vi "参数设置页.vi"() -> ()   [LabVIEW 2016, in "斯坦道总氮.lvlib"]
uses:
  <vilib>/Plasmionique/MB Master/MB_Master/MB_Master.lvclass
  <vilib>/ptbypt/NI_PtbyPt.lvlib
panel:
  in  "简易流程路径":path=path "data/流程.xml"
  out "数据刷新时间":string
  in  "通讯连接":bool
  out "MB table":enum32{"Serial", "TCP"}(tab)
  in  "请选择串口:":refnum<visa-resource-name>
  in  "IP":string="127.0.0.1"
  in  "PORT":string="1001"
  in  "通信方式选择":enum16{"串口", "TCP"}(ring)
  in  "盐度自动补偿：":bool
  out "盐度补偿值":dbl caption="盐度补偿值："
  in  "刷新":bool
  in  "测量模式":T1(ring)
  in  "参数下拉列表":u16(ring) items=["总磷"=1, "总氮"=2]
  in  "量程下拉列表":enum16{"低量程", "高量程"}(ring)
  in  "测试流程路径":path=path "data/流程.xml"
  in  "标样核查量程模式":enum16{"高量程", "低量程", "自动"}(ring) caption="标样核查量程模式："
  in  "加标回收量程模式":enum16{"高量程", "低量程", "自动"}(ring) caption="加标回收量程模式："
  in  "跨度核查量程模式":enum16{"高量程", "低量程", "自动"}(ring) caption="跨度核查量程模式："
  in  "零点核查量程模式":enum16{"高量程", "低量程", "自动"}(ring) caption="零点核查量程模式："
  in  "水样测试量程模式":enum16{"高量程", "低量程", "自动"}(ring) caption="水样测试量程模式："
  out "稀释度":dbl caption="稀释度："
  out "阈值（高->低）":dbl caption="阈值（高->低）："
  out "阈值（低->高）":dbl caption="阈值（低->高）："
  out "量程下限":dbl caption="量程下限："
  out "量程上限":dbl caption="量程上限："
  out "检出限":dbl caption="检出限："
  out "曲线截距":dbl caption="曲线截距：" format="%#.6f"
  out "曲线斜率":dbl caption="曲线斜率：" format="%#.6f"
  out "二次多项式系数":dbl caption="二次多项式系数：" format="%#.6f"
  out "消解时长":dbl caption="消解时长："
  out "消解温度":dbl caption="消解温度："
  out "测量精度":u16 caption="测量精度："
  in  "标样核查标液浓度":dbl caption="标样核查标液浓度："
  in  "跨度核查标液浓度":dbl caption="跨度核查标液浓度："
  in  "零点核查标液浓度":dbl caption="零点核查标液浓度："
  in  "跨度值":dbl caption="跨度值："
  # "ppt"
  # "mg/L"
  # "mg/L"
  # "mg/L"
  # "mg/L"
  # "mg/L"
  # "min"
  # "℃"
  # "mg/L"
  # "mg/L"
  # "mg/L"
  # "mg/L"
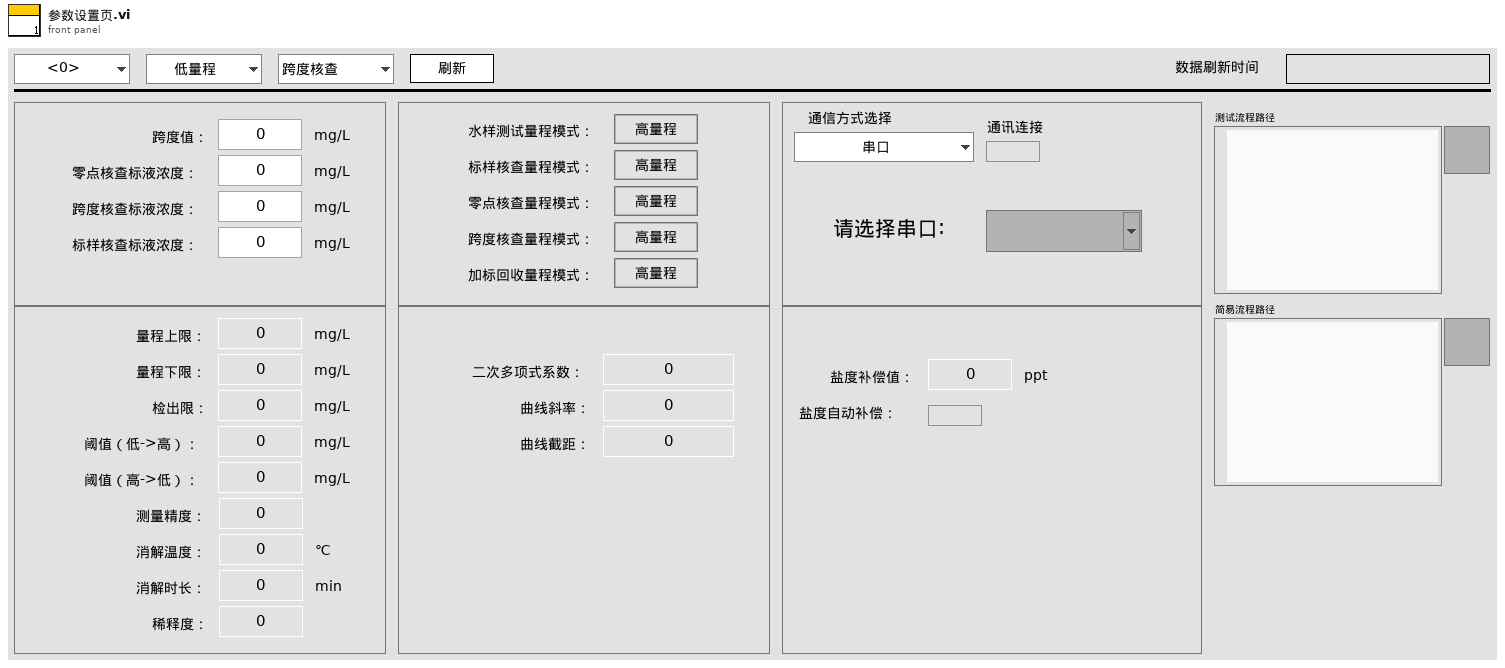
[diagram p1: front panel]
types:
  T1 = enum16{"跨度核查", "水样测量", "零点核查", "标样核查", "加标回收", "快捷测试", "空白校准", "标样校准"}
  T2 = typedef "LVStringsAndValuesArrayTypeDef_U16.ctl" = cluster{"String":string, "Value":u16}[]
  T3 = enum8{"Enabled", "Disabled", "Disabled and Grayed Out"}
  T4 = cluster{"标液浓度1":dbl, "测量吸光度1":dbl, "样品1启用":bool, "标液浓度2":dbl, "测量吸光度2":dbl, "样品2启用":bool, "标液浓度3":dbl, "测量吸光度3":dbl, "样品3启用":bool, "标液浓度4":dbl, "测量吸光度4":dbl, "样品4启用":bool, "标液浓度5":dbl, "测量吸光度5":dbl, "样品5启用":bool, "模型":enum32{"线性", "多项式"}, "精度":dbl, "XY图":cluster{"X Values":dbl[], "Y Values":dbl[]}[], "拟合公式":string, "r^2":dbl, "标样一校准时间":timestamp, "标样二校准时间":timestamp, "标样三校准时间":timestamp, "标样四校准时间":timestamp, "标样五校准时间":timestamp, "二次方程":cluster{"c":dbl, "x":dbl, "x^2":dbl}, "标定时间":timestamp}
  T5 = cluster{"系统时间":timestamp, "工作状态":u16, "测量模式":enum16{"待机", "连续模式", "周期模式", "定点模式", "受控模式", "手动模式"}, "告警代码":u16, "故障代码":u16, "日志代码":u16, "软件版本":u16, "F0":sgl, "F1":sgl, "F2":sgl, "F3":sgl, "T":sgl, "H":sgl, "id":u16, "flowid":u16, "量程":u16, "总磷控温温度1":sgl, "营养盐控温温度2":sgl, "ADC":sgl}
  T6 = cluster{"测量精度":u16, "检出限":dbl, "上限":dbl, "下限":dbl, "阈值（低->高）":dbl, "阈值（高->低）":dbl, "稀释度":dbl}
  T7 = cluster{"泵类型":u8, "进样速度":u32, "出样速度":u32, "泵阀量":u8, "光谱仪类型":u8, "光谱采样次数":u8, "氙灯次数":u8, "B":u16, "C":u16, "D":u16, "E":u16, "B_COD":u16, "C_COD":u16, "D_COD":u16, "E_COD":u16, "G":u16, "M":u16, "N":u16, "氨氮注射泵控温下限":sgl, "氨氮注射泵控温上限":sgl, "总氮注射泵控温下限":sgl, "总氮注射泵控温上限":sgl, "消解温度下限":sgl, "消解温度上限":sgl, "加热10s限值":sgl, "高温高压阀开阀温度":sgl, "总氮x公式0":u8, "总氮x公式1":sgl, "总氮x公式2":sgl, "总磷浊度稀释系数":sgl, "总磷浊度补偿权重1":sgl, "总磷浊度补偿权重2":sgl, "盐度系数":sgl, "氨氮补偿系数1":sgl, "氨氮补偿系数2":sgl}
  T8 = cluster{"标液浓度1":dbl, "测量吸光度1":dbl, "样品1启用":bool, "标液浓度2":dbl, "测量吸光度2":dbl, "样品2启用":bool, "标液浓度3":dbl, "测量吸光度3":dbl, "样品3启用":bool, "标液浓度4":dbl, "测量吸光度4":dbl, "样品4启用":bool, "标液浓度5":dbl, "测量吸光度5":dbl, "样品5启用":bool, "模型":enum32{"线性", "多项式"}, "精度":dbl, "XY图":cluster{"X Values":dbl[], "Y Values":dbl[]}[], "拟合公式":string, "r^2":dbl, "标样一校准时间":timestamp, "标样二校准时间":timestamp, "标样三校准时间":timestamp, "标样四校准时间":timestamp, "标样五校准时间":timestamp, "二次方程":cluster{"c":dbl, "x":dbl, "x^2":dbl}, "标定时间":timestamp}[][]
  T9 = typedef "斯坦道总氮.lvlib/关键参数.ctl" = cluster{"测量量程":sgl, "测量检出限":sgl, "测量精度":sgl, "测量间隔":sgl, "消解温度":sgl, "消解时长":sgl, "三项式系数":sgl, "二次多项式系数":sgl, "曲线斜率":sgl, "曲线截距":sgl, "线性相关系数":sgl, "空白校准时间":timestamp, "标样校准时间":timestamp, "测量信号值":sgl, "稀释倍数":sgl, "空白标定系数":sgl, "量程系数":sgl}
  T10 = cluster{"水样测试量程模式":enum16{"高量程", "低量程", "自动"}, "零点核查量程模式":enum16{"高量程", "低量程", "自动"}, "跨度核查量程模式":enum16{"高量程", "低量程", "自动"}, "加标回收量程模式":enum16{"高量程", "低量程", "自动"}, "标样核查量程模式":enum16{"高量程", "低量程", "自动"}}
  T11 = cluster{"总磷跨度值":dbl, "总磷零点标准液浓度":dbl, "总磷跨度标准液浓度":dbl, "总磷标准液标准浓度":dbl, "总氮跨度值":dbl, "总氮零点标准液浓度":dbl, "总氮跨度标准液浓度":dbl, "总氮标准液标准浓度":dbl, "COD跨度值":dbl, "COD零点标准液浓度":dbl, "COD跨度标准液浓度":dbl, "COD标准液标准浓度":dbl, "氨氮跨度值":dbl, "氨氮零点标准液浓度":dbl, "氨氮跨度标准液浓度":dbl, "氨氮标准液标准浓度":dbl, "磷酸盐跨度值":dbl, "磷酸盐零点标准液浓度":dbl, "磷酸盐跨度标准液浓度":dbl, "磷酸盐标准液标准浓度":dbl, "硝氮跨度值":dbl, "硝氮零点标准液浓度":dbl, "硝氮跨度标准液浓度":dbl, "硝氮标准液标准浓度":dbl, "亚硝氮跨度值":dbl, "亚硝氮零点标准液浓度":dbl, "亚硝氮跨度标准液浓度":dbl, "亚硝氮标准液标准浓度":dbl, "硫化物跨度值":dbl, "硫化物零点标准液浓度":dbl, "硫化物跨度标准液浓度":dbl, "硫化物标准液标准浓度":dbl, "硅酸盐跨度值":dbl, "硅酸盐零点标准液浓度":dbl, "硅酸盐跨度标准液浓度":dbl, "硅酸盐标准液标准浓度":dbl}
  T12 = cluster{"水样测试量程模式":u16, "零点核查量程模式":u16, "跨度核查量程模式":u16, "加标回收量程模式":u16, "标样核查量程模式":u16}
  T13 = cluster{"水样测试量程模式":enum16{"H", "L", "AUTO"}, "空白核查量程模式":enum16{"H", "L", "AUTO"}, "跨度核查量程模式":enum16{"H", "L", "AUTO"}, "加标回收量程模式":enum16{"H", "L", "AUTO"}, "标样核查量程模式":enum16{"H", "L", "AUTO"}}
  T14 = cluster{"水样测试量程模式":u16, "空白核查量程模式":u16, "跨度核查量程模式":u16, "加标回收量程模式":u16, "标样核查量程模式":u16}
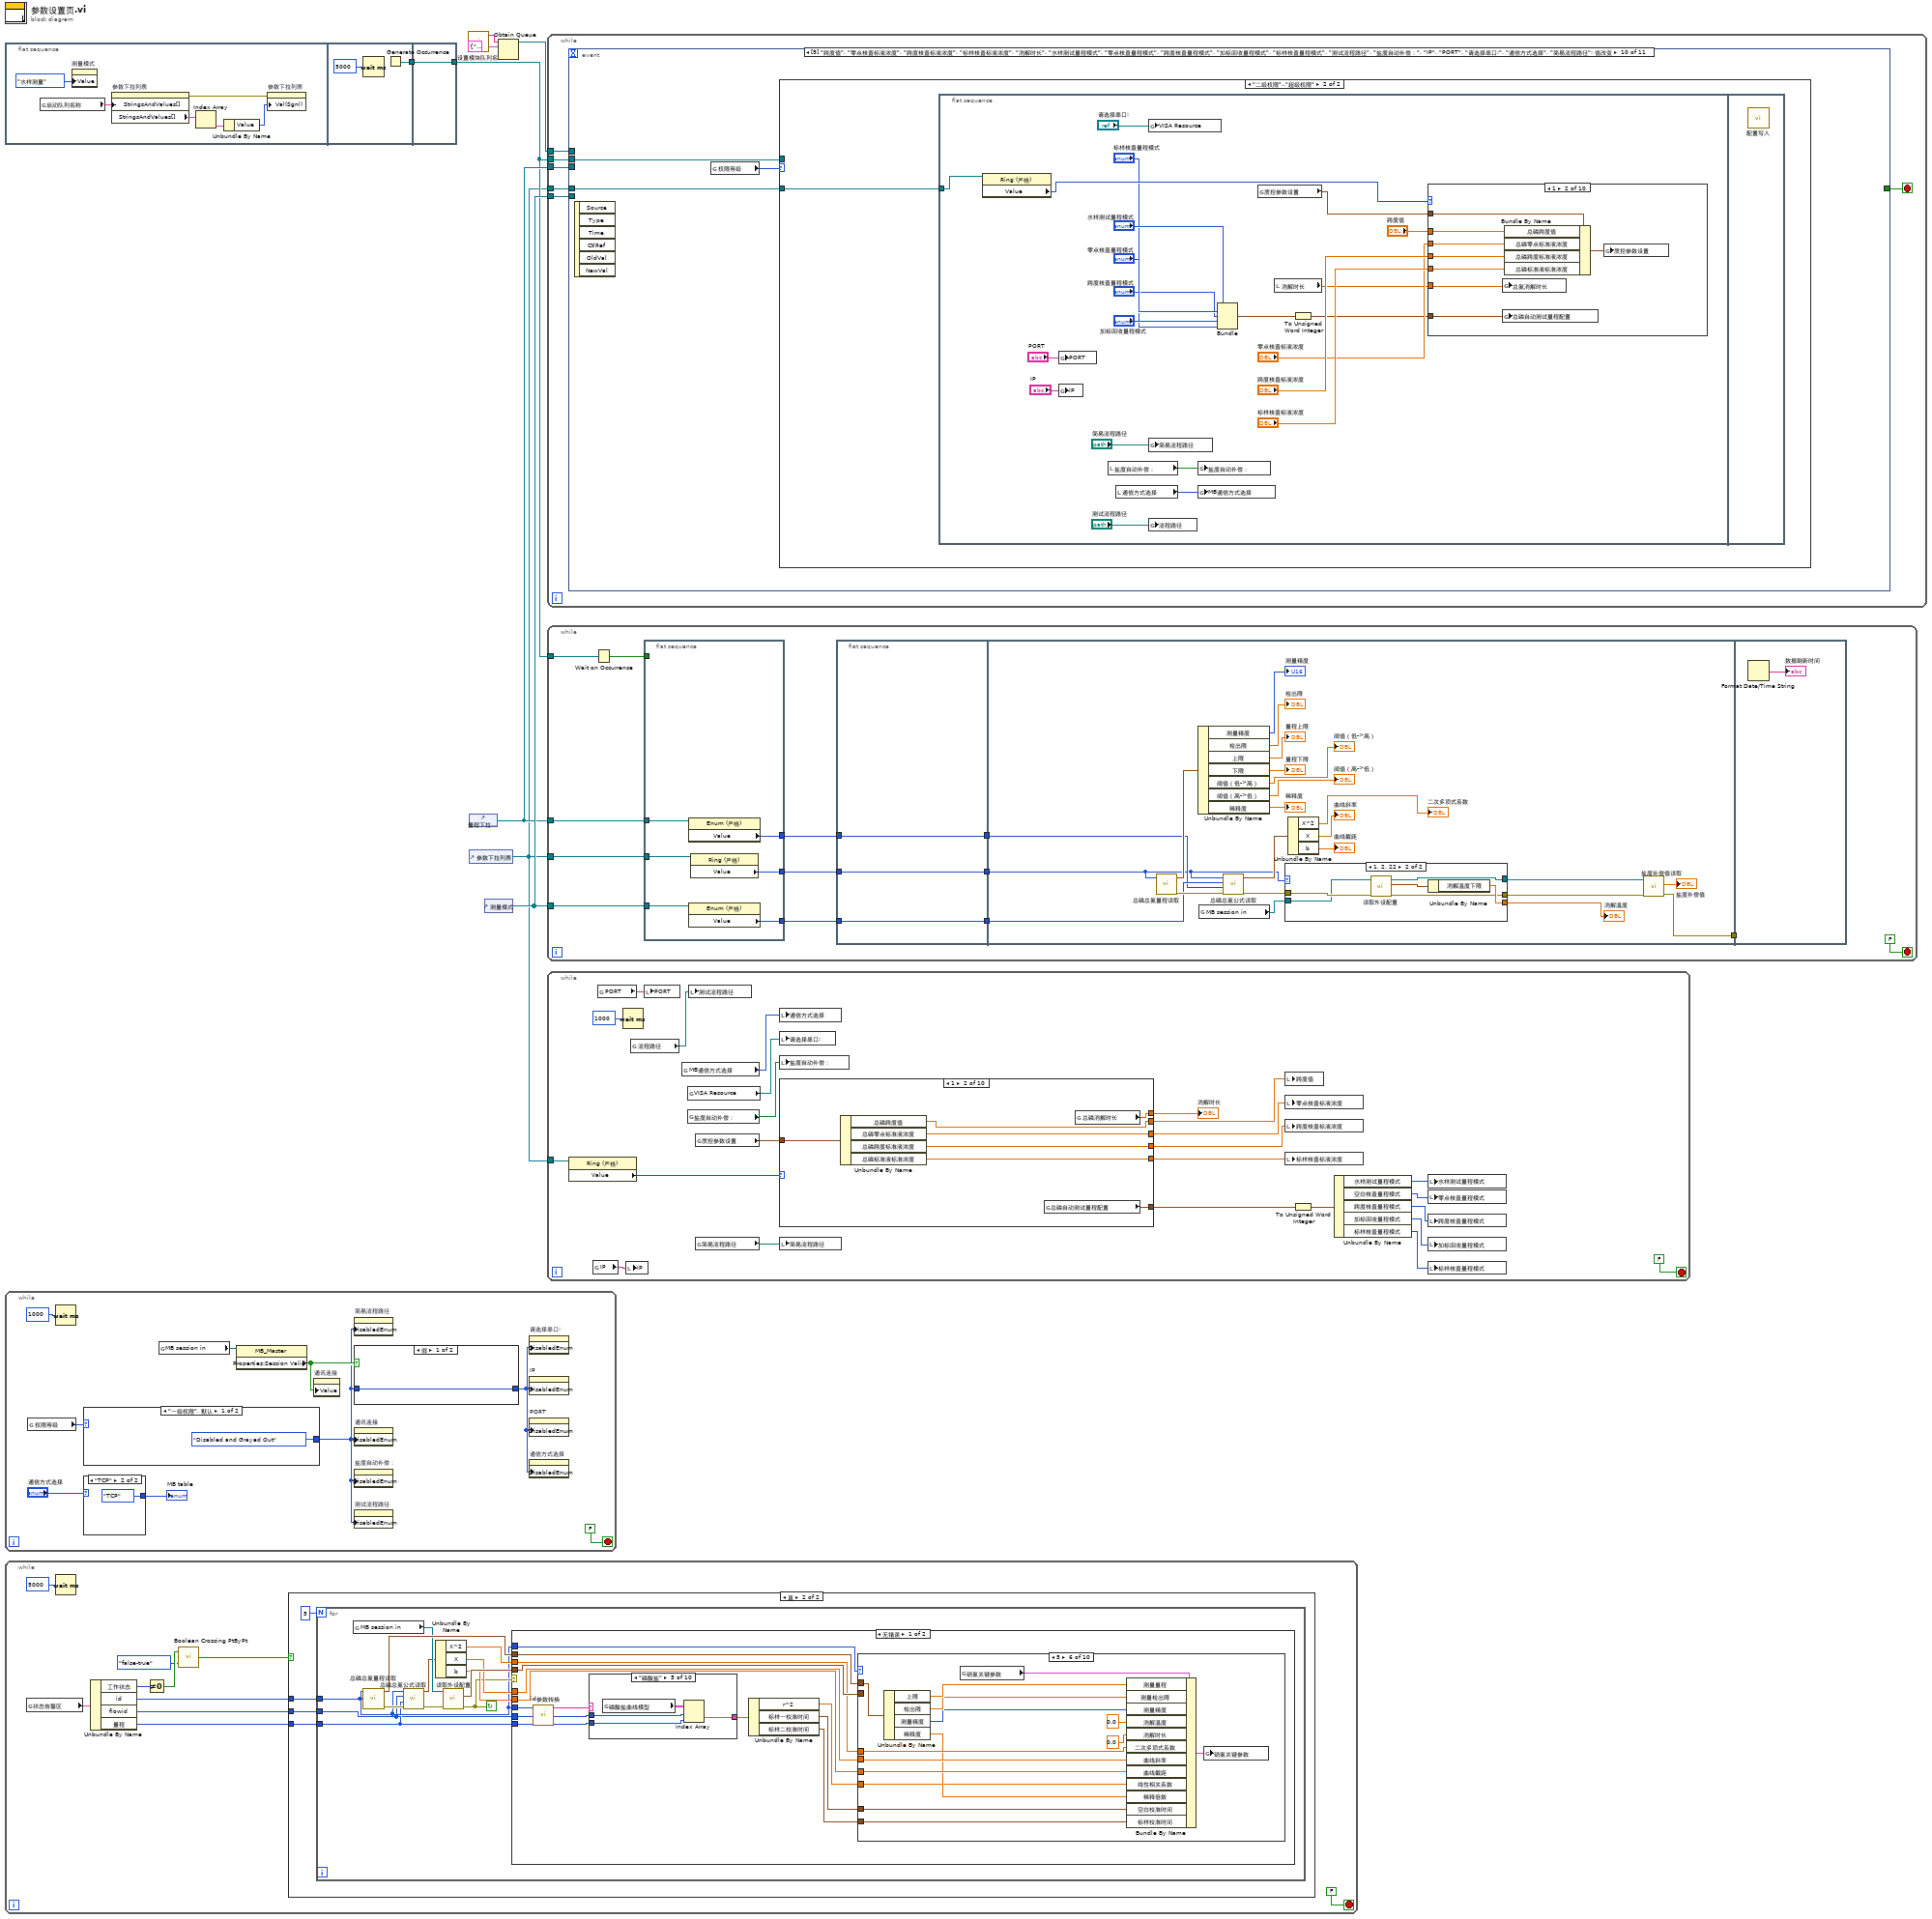
[diagram p0: block diagram]
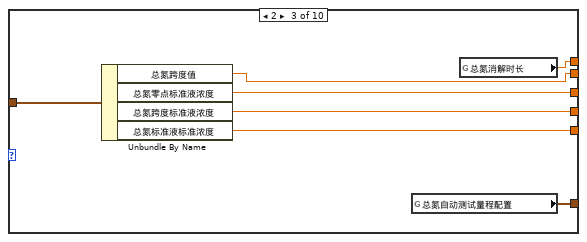
[diagram p3: hidden frame]
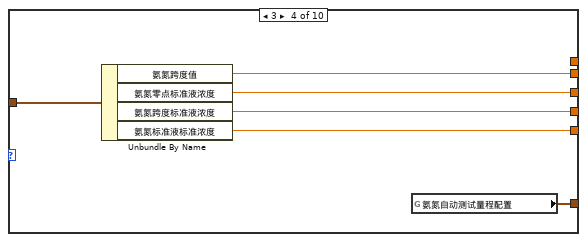
[diagram p4: hidden frame]
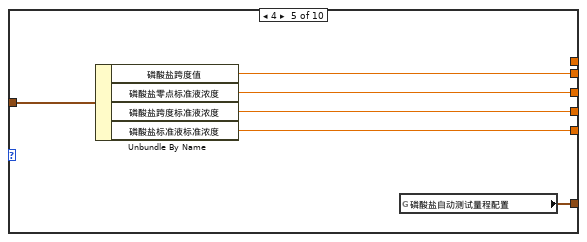
[diagram p5: hidden frame]
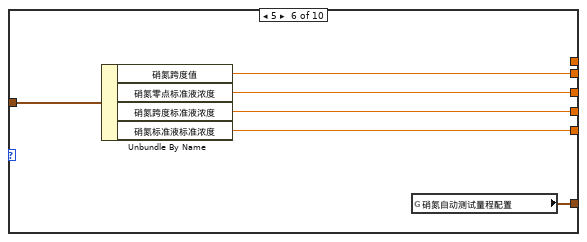
[diagram p6: hidden frame]
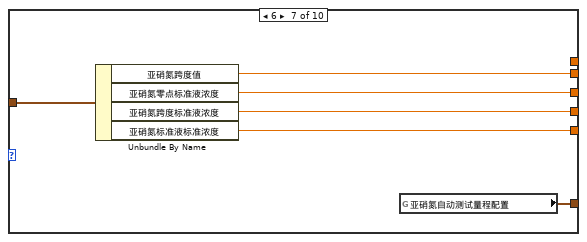
[diagram p7: hidden frame]
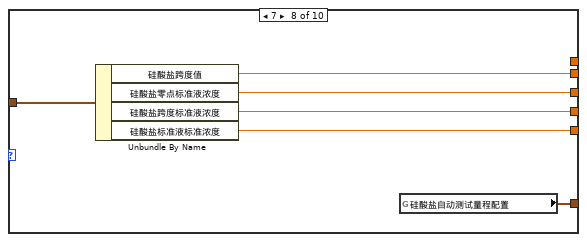
[diagram p8: hidden frame]
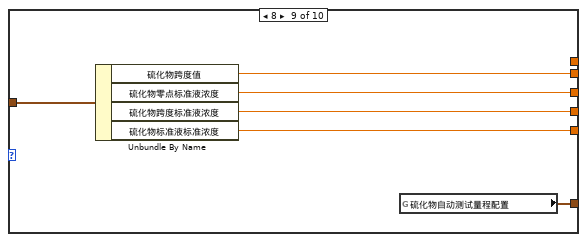
[diagram p9: hidden frame]
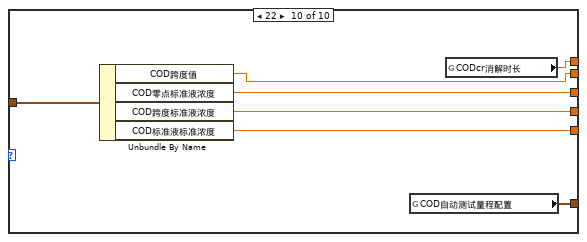
[diagram p10: hidden frame]
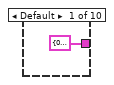
[diagram p12: hidden frame]
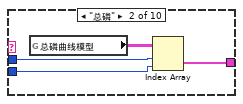
[diagram p13: hidden frame]
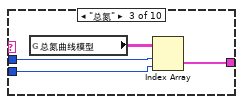
[diagram p14: hidden frame]
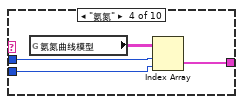
[diagram p15: hidden frame]
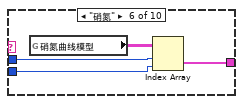
[diagram p16: hidden frame]
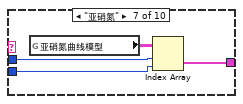
[diagram p17: hidden frame]
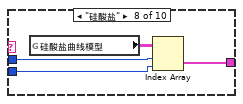
[diagram p18: hidden frame]
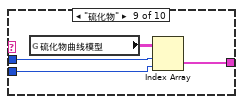
[diagram p19: hidden frame]
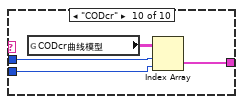
[diagram p20: hidden frame]
diagram:
  n1 = flat-sequence {
    tunnel: [w16] -> w8
    tunnel: [w17] -> w2
    tunnel: w8 -> [w17]
    frame #0 {
      n2 = global read "总磷总氮断电保存全局变量.vi" "启动队列名称"() -> (w10:cluster{"String":string, "Value":u16}[])
      n3 = property on="测量模式" class="Enum (严格)"("Value"=T1."水样测量" ("测量模式")) -> ()  [unwired: 2 in, 2 out]
      n4 = property on="参数下拉列表" class="Ring (严格)"("StringsAndValues[]"=w10) -> (error out=w13:errorcluster, "StringsAndValues[]"=w11:T2)  [unwired: 2 in, 1 out]
      n5 = Index Array(array=w11) -> (element=w12:cluster{"String":string, "Value":u16})  [unwired: 1 in]
      n6 = Unbundle By Name(w12) -> ("Value"=w14:u16)
      n7 = property on="参数下拉列表" class="Ring (严格)"(error in=w13, "Val(Sgnl)"=w14) -> ()  [unwired: 1 in, 2 out]
    }
    frame #1 {
      n8 = Wait (ms)(milliseconds to wait=u32 5000 ("等待时间（毫秒）")) -> ()  [unwired: 1 out]
      n9 = Generate Occurrence() -> (w16:refnum<k4>)
    }
    frame #2 {
    }
  }
  n10 = while {
    stop <- FALSE stop-if-true
    n11 = global read "VAR总磷总氮全局变量.vi" "权限等级"() -> (w19:enum16{"一级权限", "二级权限", "三级权限", "超级权限"})
    n12 = Wait (ms)(milliseconds to wait=u32 1000 ("等待时间（毫秒）")) -> ()  [unwired: 1 out]
    n13 = case shown="\"一级权限\", 默认" w19 {
      tunnel: [T3."Disabled and Grayed Out" ("禁用") T3."Enabled" ("禁用")] -> w18
      frame "一级权限", Default {
      }
      frame "二级权限".."超级权限" {
      }
    }
    n14 = case shown="\"TCP\"" "通信方式选择" {
      tunnel: [enum32{"Serial", "TCP"}."Serial" ("MB table") enum32{"Serial", "TCP"}."TCP" ("MB table")] -> w21
      frame "串口", Default {
      }
      frame "TCP" {
      }
    }
    "MB table" <- w21
    n15 = global read "VAR总磷总氮全局变量.vi" "MB session in"() -> (w25:refnum<class "MB_Master.lvclass">)
    n16 = property class="MB_Master"(reference=w25) -> ("Properties:Session Valid"=w23:bool)  [unwired: 1 in, 2 out]
    n17 = property on="通讯连接" class="Bool (严格)"("Value"=w23) -> ()  [unwired: 2 in, 2 out]
    n18 = property on="简易流程路径" class="Path"("DisabledEnum"=w18) -> ()  [unwired: 2 in, 2 out]
    n19 = case shown="假" w23 {
      tunnel: [w31 T3."Disabled and Grayed Out" ("禁用")] -> w22
      tunnel: w18 -> [w31 _]
      frame False {
      }
      frame True {
      }
    }
    n20 = property on="通讯连接" class="Bool (严格)"("DisabledEnum"=w18) -> ()  [unwired: 2 in, 2 out]
    n21 = property on="盐度自动补偿：" class="Bool (严格)"("DisabledEnum"=w18) -> ()  [unwired: 2 in, 2 out]
    n22 = property on="测试流程路径" class="Path"("DisabledEnum"=w18) -> ()  [unwired: 2 in, 2 out]
    n23 = property on="请选择串口:" class="VISAName"("DisabledEnum"=w22) -> ()  [unwired: 2 in, 2 out]
    n24 = property on="IP" class="Str"("DisabledEnum"=w22) -> ()  [unwired: 2 in, 2 out]
    n25 = property on="PORT" class="Str"("DisabledEnum"=w22) -> ()  [unwired: 2 in, 2 out]
    n26 = property on="通信方式选择" class="Enum (严格)"("DisabledEnum"=w22) -> ()  [unwired: 2 in, 2 out]
  }
  n27 = while {
    stop <- FALSE stop-if-true
    n28 = global read "VAR总磷总氮全局变量.vi" "状态告警区"() -> (w42:T5)
    n29 = Wait (ms)(milliseconds to wait=u32 5000 ("等待时间（毫秒）")) -> ()  [unwired: 1 out]
    n30 = Unbundle By Name(w42) -> ("工作状态"=w38:u16, "id"=w39:u16, "flowid"=w40:u16, "量程"=w41:u16)
    n31 = Not Equal To 0?(x=w38) -> (x != 0?=w37:bool)
    n32 = call <vilib>:"Boolean Crossing PtByPt.vi"("direction"=enum16{"either", "false-true", "true-false"}."false-true", "input"=w37) -> ("crossing"=w35:bool)  [unwired: 1 in]
    n33 = case shown="真" w35 {
      tunnel: w41 -> [_ w46]
      tunnel: w40 -> [_ w45]
      tunnel: w39 -> [_ w44]
      frame False {
      }
      frame True {
        n34 = for {
          N: 5 -> [_]
          tunnel: w46 -> [w48]
          tunnel: w45 -> [w47]
          tunnel: w44 -> [w49]
          stop <- w50 continue-if-true
          n35 = global read "VAR总磷总氮全局变量.vi" "MB session in"() -> (w58:refnum<class "MB_Master.lvclass">)
          n36 = call "总磷总氮量程读取.vi"("测量参数"=w49) -> ("error out"=w52:errorcluster, "量程参数读取"=w59:T6)  [unwired: 9 in]
          n37 = call "总磷总氮公式读取.vi"("error in (no error)"=w52, "量程"=w48, "测量模式"=w47, "测量参数"=w49) -> ("error out"=w51:errorcluster, "公式"=w56:cluster{"X^2":dbl, "X":dbl, "b":dbl})  [unwired: 6 in]
          n38 = Unbundle By Name(w56) -> ("X^2"=w55:dbl, "X"=w54:dbl, "b"=w53:dbl)
          n39 = call "读取外设配置.vi"("error in (no error)"=w51, "MB session in"=w58) -> ("error out"=w50:errorcluster, "外设配置"=w57:T7)  [unwired: 7 in, 1 out]
          n40 = case shown="无错误" w50 {
            tunnel: w59 -> [w73 _]
            tunnel: w57 -> [w72 _]
            tunnel: w55 -> [w71 _]
            tunnel: w54 -> [w70 _]
            tunnel: w53 -> [w69 _]
            tunnel: w49 -> [w68 _]
            tunnel: w49 -> [w65 _]
            tunnel: w48 -> [w61 _]
            tunnel: w47 -> [w60 _]
            frame No Error {
              n41 = call "id参数转换.vi"("id"=w65) -> ("table输出"=w67:string)  [unwired: 9 in, 1 out]
              n42 = case shown="\"磷酸盐\"" w67 {
                tunnel: w61 -> [_ w77 w79 w84 w88 w92 w96 w100 w104 w108]
                tunnel: w60 -> [_ w78 w80 w85 w89 w93 w97 w101 w105 w109]
                tunnel: [T4 {"标液浓度1"=0.0, "测量吸光度1"=0.0, "样品1启用"=FALSE, "标液浓度2"=0.0, "测量吸光度2"=0.0, "样品2启用"=FALSE, "标液浓度3"=0.0, "测量吸光度3"=0.0, "样品3启用"=FALSE, "标液浓度4"=0.0, "测量吸光度4"=0.0, "样品4启用"=FALSE, "标液浓度5"=0.0, "测量吸光度5"=0.0, "样品5启用"=FALSE, "模型"=enum."线性", "精度"=0.0, "XY图"=[], "拟合公式"="", "r^2"=0.0, "标样一校准时间"=timestamp(0 s since 1904-01-01), "标样二校准时间"=timestamp(0 s since 1904-01-01), "标样三校准时间"=timestamp(0 s since 1904-01-01), "标样四校准时间"=timestamp(0 s since 1904-01-01), "标样五校准时间"=timestamp(0 s since 1904-01-01), "二次方程"={"c"=0.0, "x"=0.0, "x^2"=0.0}, "标定时间"=timestamp(0 s since 1904-01-01)} ("总磷曲线模型") w75 w81 w83 w87 w91 w95 w99 w103 w107] -> w66
                frame Default {
                }
                frame "总磷" {
                  n43 = global read "校准数据全局变量.vi" "总磷曲线模型"() -> (w76:T8)
                  n44 = Index Array(array=w76, index (row)=w78, index (col)=w77) -> (element=w75:T4)
                }
                frame "总氮" {
                  n45 = global read "校准数据全局变量.vi" "总氮曲线模型"() -> (w82:T8)
                  n46 = Index Array(array=w82, index (row)=w80, index (col)=w79) -> (element=w81:T4)
                }
                frame "氨氮" {
                  n47 = global read "校准数据全局变量.vi" "氨氮曲线模型"() -> (w86:T8)
                  n48 = Index Array(array=w86, index (row)=w85, index (col)=w84) -> (element=w83:T4)
                }
                frame "磷酸盐" {
                  n49 = global read "校准数据全局变量.vi" "磷酸盐曲线模型"() -> (w90:T8)
                  n50 = Index Array(array=w90, index (row)=w89, index (col)=w88) -> (element=w87:T4)
                }
                frame "硝氮" {
                  n51 = global read "校准数据全局变量.vi" "硝氮曲线模型"() -> (w94:T8)
                  n52 = Index Array(array=w94, index (row)=w93, index (col)=w92) -> (element=w91:T4)
                }
                frame "亚硝氮" {
                  n53 = global read "校准数据全局变量.vi" "亚硝氮曲线模型"() -> (w98:T8)
                  n54 = Index Array(array=w98, index (row)=w97, index (col)=w96) -> (element=w95:T4)
                }
                frame "硅酸盐" {
                  n55 = global read "校准数据全局变量.vi" "硅酸盐曲线模型"() -> (w102:T8)
                  n56 = Index Array(array=w102, index (row)=w101, index (col)=w100) -> (element=w99:T4)
                }
                frame "硫化物" {
                  n57 = global read "校准数据全局变量.vi" "硫化物曲线模型"() -> (w106:T8)
                  n58 = Index Array(array=w106, index (row)=w105, index (col)=w104) -> (element=w103:T4)
                }
                frame "CODcr" {
                  n59 = global read "校准数据全局变量.vi" "CODcr曲线模型"() -> (w110:T8)
                  n60 = Index Array(array=w110, index (row)=w109, index (col)=w108) -> (element=w107:T4)
                }
              }
              n61 = Unbundle By Name(w66) -> ("r^2"=w64:dbl, "标样一校准时间"=w63:timestamp, "标样二校准时间"=w62:timestamp)
              n62 = case shown="5" w68 {
                tunnel: w73 -> [_ w124 w140 w155 w170 w185 w198 w213 w228 w244]
                tunnel: w72 -> [_ w120 w136 _ _ _ _ _ _ w236]
                tunnel: w71 -> [_ w117 w133 w151 w166 w181 w194 w209 w224 w240]
                tunnel: w70 -> [_ w116 w132 w150 w165 w180 w193 w208 w223 w239]
                tunnel: w69 -> [_ w115 w131 w149 w164 w179 w192 w207 w222 w238]
                tunnel: w64 -> [_ w111 w129 w145 w158 w175 _ w203 w216 w233]
                tunnel: w63 -> [_ w112 w128 w144 w160 w174 _ w202 w218 w232]
                tunnel: w62 -> [_ w113 w127 w143 w159 w173 _ w201 w217 w231]
                frame 0, Default {
                }
                frame 1 {
                  n63 = Unbundle By Name(w120) -> ("消解温度下限"=w119:sgl)
                  n64 = Unbundle By Name(w124) -> ("上限"=w123:dbl, "检出限"=w122:dbl, "测量精度"=w121:u16, "稀释度"=w114:dbl)
                  n65 = global read "VAR总磷总氮全局变量.vi" "总磷关键参数"() -> (w125:T9)
                  n66 = global read "总磷总氮断电保存全局变量.vi" "总磷消解时长"() -> (w118:dbl)
                  n67 = Bundle By Name(cluster=w125, "测量量程"=w123, "测量检出限"=w122, "测量精度"=w121, "消解温度"=w119, "消解时长"=w118, "二次多项式系数"=w117, "曲线斜率"=w116, "曲线截距"=w115, "线性相关系数"=w111, "稀释倍数"=w114, "空白校准时间"=w112, "标样校准时间"=w113) -> (w126:T9)
                  n68 = global write "VAR总磷总氮全局变量.vi" "总磷关键参数"(w126) -> ()
                }
                frame 2 {
                  n69 = Unbundle By Name(w136) -> ("消解温度下限"=w135:sgl)
                  n70 = Unbundle By Name(w140) -> ("上限"=w139:dbl, "检出限"=w138:dbl, "测量精度"=w137:u16, "稀释度"=w130:dbl)
                  n71 = global read "VAR总磷总氮全局变量.vi" "总氮关键参数"() -> (w141:T9)
                  n72 = global read "总磷总氮断电保存全局变量.vi" "总氮消解时长"() -> (w134:dbl)
                  n73 = Bundle By Name(cluster=w141, "测量量程"=w139, "测量检出限"=w138, "测量精度"=w137, "消解温度"=w135, "消解时长"=w134, "二次多项式系数"=w133, "曲线斜率"=w132, "曲线截距"=w131, "线性相关系数"=w129, "稀释倍数"=w130, "空白校准时间"=w128, "标样校准时间"=w127) -> (w142:T9)
                  n74 = global write "VAR总磷总氮全局变量.vi" "总氮关键参数"(w142) -> ()
                }
                frame 3 {
                  n75 = Unbundle By Name(w155) -> ("上限"=w154:dbl, "检出限"=w153:dbl, "测量精度"=w152:u16, "稀释度"=w148:dbl)
                  n76 = global read "VAR总磷总氮全局变量.vi" "氨氮关键参数"() -> (w156:T9)
                  n77 = Bundle By Name(cluster=w156, "测量量程"=w154, "测量检出限"=w153, "测量精度"=w152, "消解温度"=sgl 0.0, "消解时长"=sgl 0.0, "二次多项式系数"=w151, "曲线斜率"=w150, "曲线截距"=w149, "线性相关系数"=w145, "稀释倍数"=w148, "空白校准时间"=w144, "标样校准时间"=w143) -> (w157:T9)
                  n78 = global write "VAR总磷总氮全局变量.vi" "氨氮关键参数"(w157) -> ()
                }
                frame 4 {
                  n79 = Unbundle By Name(w170) -> ("上限"=w169:dbl, "检出限"=w168:dbl, "测量精度"=w167:u16, "稀释度"=w163:dbl)
                  n80 = global read "VAR总磷总氮全局变量.vi" "磷酸盐关键参数"() -> (w171:T9)
                  n81 = Bundle By Name(cluster=w171, "测量量程"=w169, "测量检出限"=w168, "测量精度"=w167, "消解温度"=sgl 0.0, "消解时长"=sgl 0.0, "二次多项式系数"=w166, "曲线斜率"=w165, "曲线截距"=w164, "线性相关系数"=w158, "稀释倍数"=w163, "空白校准时间"=w160, "标样校准时间"=w159) -> (w172:T9)
                  n82 = global write "VAR总磷总氮全局变量.vi" "磷酸盐关键参数"(w172) -> ()
                }
                frame 5 {
                  n83 = Unbundle By Name(w185) -> ("上限"=w184:dbl, "检出限"=w183:dbl, "测量精度"=w182:u16, "稀释度"=w178:dbl)
                  n84 = global read "VAR总磷总氮全局变量.vi" "硝氮关键参数"() -> (w186:T9)
                  n85 = Bundle By Name(cluster=w186, "测量量程"=w184, "测量检出限"=w183, "测量精度"=w182, "消解温度"=sgl 0.0, "消解时长"=sgl 0.0, "二次多项式系数"=w181, "曲线斜率"=w180, "曲线截距"=w179, "线性相关系数"=w175, "稀释倍数"=w178, "空白校准时间"=w174, "标样校准时间"=w173) -> (w187:T9)
                  n86 = global write "VAR总磷总氮全局变量.vi" "硝氮关键参数"(w187) -> ()
                }
                frame 6 {
                  n87 = Unbundle By Name(w198) -> ("上限"=w197:dbl, "检出限"=w196:dbl, "测量精度"=w195:u16, "稀释度"=w190:dbl)
                  n88 = global read "VAR总磷总氮全局变量.vi" "亚硝氮关键参数"() -> (w199:T9)
                  n89 = Bundle By Name(cluster=w199, "测量量程"=w197, "测量检出限"=w196, "测量精度"=w195, "消解温度"=sgl 0.0, "消解时长"=sgl 0.0, "二次多项式系数"=w194, "曲线斜率"=w193, "曲线截距"=w192, "线性相关系数"=sgl 1.0, "稀释倍数"=w190) -> (w200:T9)
                  n90 = global write "VAR总磷总氮全局变量.vi" "亚硝氮关键参数"(w200) -> ()
                }
                frame 7 {
                  n91 = Unbundle By Name(w213) -> ("上限"=w212:dbl, "检出限"=w211:dbl, "测量精度"=w210:u16, "稀释度"=w206:dbl)
                  n92 = global read "VAR总磷总氮全局变量.vi" "硅酸盐关键参数"() -> (w214:T9)
                  n93 = Bundle By Name(cluster=w214, "测量量程"=w212, "测量检出限"=w211, "测量精度"=w210, "消解温度"=sgl 0.0, "消解时长"=sgl 0.0, "二次多项式系数"=w209, "曲线斜率"=w208, "曲线截距"=w207, "线性相关系数"=w203, "稀释倍数"=w206, "空白校准时间"=w202, "标样校准时间"=w201) -> (w215:T9)
                  n94 = global write "VAR总磷总氮全局变量.vi" "硅酸盐关键参数"(w215) -> ()
                }
                frame 8 {
                  n95 = Unbundle By Name(w228) -> ("上限"=w227:dbl, "检出限"=w226:dbl, "测量精度"=w225:u16, "稀释度"=w221:dbl)
                  n96 = global read "VAR总磷总氮全局变量.vi" "硫化物关键参数"() -> (w229:T9)
                  n97 = Bundle By Name(cluster=w229, "测量量程"=w227, "测量检出限"=w226, "测量精度"=w225, "消解温度"=sgl 0.0, "消解时长"=sgl 0.0, "二次多项式系数"=w224, "曲线斜率"=w223, "曲线截距"=w222, "线性相关系数"=w216, "稀释倍数"=w221, "空白校准时间"=w218, "标样校准时间"=w217) -> (w230:T9)
                  n98 = global write "VAR总磷总氮全局变量.vi" "硫化物关键参数"(w230) -> ()
                }
                frame 22 {
                  n99 = Unbundle By Name(w236) -> ("消解温度下限"=w235:sgl)
                  n100 = Unbundle By Name(w244) -> ("上限"=w243:dbl, "检出限"=w242:dbl, "测量精度"=w241:u16, "稀释度"=w237:dbl)
                  n101 = global read "VAR总磷总氮全局变量.vi" "CODcr关键参数"() -> (w245:T9)
                  n102 = global read "总磷总氮断电保存全局变量.vi" "CODcr消解时长"() -> (w234:dbl)
                  n103 = Bundle By Name(cluster=w245, "测量量程"=w243, "测量检出限"=w242, "测量精度"=w241, "消解温度"=w235, "消解时长"=w234, "二次多项式系数"=w240, "曲线斜率"=w239, "曲线截距"=w238, "线性相关系数"=w233, "稀释倍数"=w237, "空白校准时间"=w232, "标样校准时间"=w231) -> (w246:T9)
                  n104 = global write "VAR总磷总氮全局变量.vi" "CODcr关键参数"(w246) -> ()
                }
              }
            }
            frame Error {
            }
          }
        }
      }
    }
  }
  n105 = call "设置模块队列名.vi"() -> ("Msg"=w6:string)  [unwired: 5 in]
  n106 = control-ref of="量程下拉列表"() -> (w3:refnum<vi>)
  n107 = control-ref of="参数下拉列表"() -> (w1:refnum<vi>)
  n108 = control-ref of="测量模式"() -> (w4:refnum<vi>)
  n109 = Obtain Queue(name (unnamed)=w6, element data type=cluster{"命令":string, "data":variant} {"命令"="", "data"=variant}) -> (queue out=w5:refnum<queue>)  [unwired: 3 in, 2 out]
  n110 = while {
    tunnel: w2 -> [w251]
    tunnel: w1 -> [w250]
    tunnel: w5 -> [w249]
    tunnel: w4 -> [w248]
    tunnel: w3 -> [w247]
    stop <- w252 stop-if-true
    n111 = event shown="[9] \"跨度值\", \"零点核查标液浓度\", \"跨度核查标液浓度\", \"标样核查标液浓度\", \"消解时长\", \"水样测试量程模式\", \"零点核查量程模式\", \"跨度核查量程模式\", \"加标回收量程模式\", \"标样核查量程模式\", \"测试流程路径\", \"盐度自动补偿：\", \"IP\", \"PORT\", \"请选择串口:\", \"通信方式选择\", \"简易流程路径\": 值改变" {
      selector: _ -> [_ _ _ _ _ _ _ _ _ _ _]
      dyn-events: _ -> [_ _ _ _ _ _ _ _ _ _ _]
      timeout: _ -> [_ _ _ _ _ _ _ _ _ _ _]
      tunnel: [_ TRUE _ _ _ _ _ _ _ _ _] -> w252
      tunnel: w251 -> [_ _ w254 _ _ _ _ _ _ w301 _]
      tunnel: w250 -> [_ _ _ _ w273 _ _ _ _ w303 _]
      tunnel: w249 -> [_ _ _ _ _ _ _ _ _ _ w394]
      tunnel: w248 -> [_ _ _ _ _ _ _ _ _ _ _]
      tunnel: w247 -> [_ _ _ _ _ _ _ _ _ _ _]
      event Timeout {
        n112 = event-data() -> ()  [unwired: 1 in, 3 out]
      }
      event Panel Close {
        n113 = event-data() -> ()  [unwired: 1 in, 4 out]
      }
      event "参数下拉列表", "量程下拉列表", "测量模式", "刷新": Value Change {
        n114 = event-data() -> ()  [unwired: 1 in, 6 out]
        n115 = Set Occurrence(w254) -> ()
      }
      event "跨度值", "零点核查标液浓度", "跨度核查标液浓度", "标样核查标液浓度", "消解温度", "消解时长", "检出限", "量程上限", "量程下限", "阈值（低->高）", "阈值（高->低）", "稀释度": Mouse Down {
        n116 = event-data() -> ("CtlRef"=w256:refnum<vi>)  [unwired: 1 in, 5 out]
        n117 = global read "VAR总磷总氮全局变量.vi" "权限等级"() -> (w255:enum16{"一级权限", "二级权限", "三级权限", "超级权限"})
        n118 = case shown="\"二级权限\"..\"超级权限\"" w255 {
          tunnel: w256 -> [_ w260]
          frame "一级权限", Default {
          }
          frame "二级权限".."超级权限" {
            n119 = property class="DigNum (严格)"(reference=w260) -> (reference out=w258:refnum<vi>, "Value"=w259:dbl)  [unwired: 1 in, 1 out]
            n120 = call "数字键盘.vi"("OldNumber"=w259) -> ("NewNumber"=w257:dbl)
            n121 = property class="DigNum (严格)"(reference=w258, "Val(Sgnl)"=w257) -> ()  [unwired: 1 in, 2 out]
          }
        }
      }
      event "测量精度", "检出限", "量程上限", "量程下限", "阈值（低->高）", "阈值（高->低）", "稀释度": Value Change {
        n122 = event-data() -> ()  [unwired: 1 in, 6 out]
        n123 = property class="Ring (严格)"(reference=w273) -> ("Value"=w272:u16)  [unwired: 1 in, 2 out]
        n124 = local read "阈值（低->高）"() -> (w266:dbl)
        n125 = local read "阈值（高->低）"() -> (w265:dbl)
        n126 = local read "测量精度"() -> (w263:u16)
        n127 = local read "量程下限"() -> (w268:dbl)
        n128 = local read "量程上限"() -> (w269:dbl)
        n129 = local read "稀释度"() -> (w264:dbl)
        n130 = local read "检出限"() -> (w267:dbl)
        n131 = Bundle By Name(cluster=T6 {"测量精度"=0, "检出限"=0.0, "上限"=0.0, "下限"=0.0, "阈值（低->高）"=0.0, "阈值（高->低）"=0.0, "稀释度"=0.0} ("量程参数写入"), "测量精度"=w263, "检出限"=w267, "上限"=w269, "下限"=w268, "阈值（低->高）"=w266, "阈值（高->低）"=w265, "稀释度"=w264) -> (w270:T6)
        n132 = call "总磷总氮量程写入.vi"("量程参数写入"=w270, "测量参数"=w272) -> ("error out"=w261:errorcluster)  [unwired: 8 in]
        n133 = case shown="错误" w261 {
          tunnel: ["写入成功" "写入失败"] -> w262
          frame No Error {
          }
          frame Error {
          }
        }
        n134 = One Button Dialog(message=w262) -> ()  [unwired: 1 in, 1 out]
      }
      event "消解温度": Value Change {
        n135 = event-data() -> ("NewVal"=w278:dbl)  [unwired: 1 in, 5 out]
        n136 = global read "VAR总磷总氮全局变量.vi" "MB session in"() -> (w279:refnum<class "MB_Master.lvclass">)
        n137 = call "读取外设配置.vi"("MB session in"=w279) -> ("error out"=w282:errorcluster, "外设配置"=w281:T7)  [unwired: 8 in, 1 out]
        n138 = Bundle By Name(cluster=w281, "消解温度下限"=w278) -> (w280:T7)
        n139 = call "写入外设配置.vi"("error in (no error)"=w282, "外设配置"=w280, "MB session in"=w279) -> ("error out"=w277:errorcluster)  [unwired: 7 in, 1 out]
        n140 = case shown="错误" w277 {
          tunnel: ["写入成功" "写入失败"] -> w276
          frame No Error {
          }
          frame Error {
          }
        }
        n141 = One Button Dialog(message=w276) -> ()  [unwired: 1 in, 1 out]
      }
      event "测量精度": Mouse Down {
        n142 = event-data() -> ("CtlRef"=w286:refnum<vi>)  [unwired: 1 in, 7 out]
        n143 = global read "VAR总磷总氮全局变量.vi" "权限等级"() -> (w285:enum16{"一级权限", "二级权限", "三级权限", "超级权限"})
        n144 = case shown="\"二级权限\"..\"超级权限\"" w285 {
          tunnel: w286 -> [_ w290]
          frame "一级权限", Default {
          }
          frame "二级权限".."超级权限" {
            n145 = property class="DigNum (严格)"(reference=w290) -> (reference out=w288:refnum<vi>, "Value"=w289:u16)  [unwired: 1 in, 1 out]
            n146 = call "数字键盘.vi"("OldNumber"=w289) -> ("NewNumber"=w287:dbl)
            n147 = property class="DigNum (严格)"(reference=w288, "Val(Sgnl)"=w287) -> ()  [unwired: 1 in, 2 out]
          }
        }
      }
      event "盐度补偿值": Mouse Down {
        n148 = event-data() -> ("CtlRef"=w292:refnum<vi>)  [unwired: 1 in, 3 out]
        n149 = global read "VAR总磷总氮全局变量.vi" "权限等级"() -> (w291:enum16{"一级权限", "二级权限", "三级权限", "超级权限"})
        n150 = case shown="\"二级权限\"..\"超级权限\"" w291 {
          tunnel: w292 -> [_ w294]
          frame "一级权限", Default {
          }
          frame "二级权限".."超级权限" {
            n151 = case shown="假" "盐度自动补偿：" {
              tunnel: w294 -> [w298 _]
              frame False {
                n152 = property class="DigNum (严格)"(reference=w298) -> (reference out=w296:refnum<vi>, "Value"=w297:dbl)  [unwired: 1 in, 1 out]
                n153 = call "数字键盘.vi"("OldNumber"=w297) -> ("NewNumber"=w295:dbl)
                n154 = property class="DigNum (严格)"(reference=w296, "Val(Sgnl)"=w295) -> ()  [unwired: 1 in, 2 out]
              }
              frame True {
              }
            }
          }
        }
      }
      event "盐度补偿值": Value Change {
        n155 = event-data() -> ("NewVal"=w299:dbl)  [unwired: 1 in, 5 out]
        n156 = global read "VAR总磷总氮全局变量.vi" "MB session in"() -> (w300:refnum<class "MB_Master.lvclass">)
        n157 = call "盐度补偿值写入.vi"("盐度补偿值"=w299, "MB session in"=w300) -> ()  [unwired: 8 in, 2 out]
      }
      event "跨度值", "零点核查标液浓度", "跨度核查标液浓度", "标样核查标液浓度", "消解时长", "水样测试量程模式", "零点核查量程模式", "跨度核查量程模式", "加标回收量程模式", "标样核查量程模式", "测试流程路径", "盐度自动补偿：", "IP", "PORT", "请选择串口:", "通信方式选择", "简易流程路径": Value Change {
        n158 = event-data() -> ()  [unwired: 1 in, 6 out]
        n159 = global read "VAR总磷总氮全局变量.vi" "权限等级"() -> (w302:enum16{"一级权限", "二级权限", "三级权限", "超级权限"})
        n160 = case shown="\"二级权限\"..\"超级权限\"" w302 {
          tunnel: w303 -> [_ w305]
          tunnel: w301 -> [w304 _]
          frame "一级权限", Default {
            n161 = Set Occurrence(w304) -> ()
          }
          frame "二级权限".."超级权限" {
            n162 = flat-sequence {
              tunnel: w305 -> [w326]
              frame #0 {
                n163 = property class="Ring (严格)"(reference=w326) -> ("Value"=w325:u16)  [unwired: 1 in, 2 out]
                n164 = global write "总磷总氮断电保存全局变量.vi" "PORT"("PORT") -> ()
                n165 = global write "总磷总氮断电保存全局变量.vi" "IP"("IP") -> ()
                n166 = local read "盐度自动补偿："() -> (w312:bool)
                n167 = local read "通信方式选择"() -> (w308:enum16{"串口", "TCP"})
                n168 = global write "总磷总氮断电保存全局变量.vi" "VISA Resource"("请选择串口:") -> ()
                n169 = global write "总磷总氮断电保存全局变量.vi" "简易流程路径"("简易流程路径") -> ()
                n170 = global write "总磷总氮断电保存全局变量.vi" "流程路径"("测试流程路径") -> ()
                n171 = global write "总磷总氮断电保存全局变量.vi" "盐度自动补偿："(w312) -> ()
                n172 = global write "总磷总氮断电保存全局变量.vi" "MB通信方式选择"(w308) -> ()
                n173 = Bundle("水样测试量程模式"="水样测试量程模式", "零点核查量程模式"="零点核查量程模式", "跨度核查量程模式"="跨度核查量程模式", "加标回收量程模式"="加标回收量程模式", "标样核查量程模式"="标样核查量程模式") -> (w314:T10)  [unwired: 1 in]
                n174 = global read "总磷总氮断电保存全局变量.vi" "质控参数设置"() -> (w320:T11)
                n175 = local read "消解时长"() -> (w307:dbl)
                n176 = To Unsigned Word Integer(number=w314) -> (unsigned 16bit integer=w313:T12)
                n177 = case shown="1" w325 {
                  tunnel: "跨度值" -> [_ w333 w341 w348 w355 w362 w369 w376 w383 w390]
                  tunnel: "标样核查标液浓度" -> [_ w330 w338 w345 w352 w359 w366 w373 w380 w387]
                  tunnel: "跨度核查标液浓度" -> [_ w331 w339 w346 w353 w360 w367 w374 w381 w388]
                  tunnel: "零点核查标液浓度" -> [_ w332 w340 w347 w354 w361 w368 w375 w382 w389]
                  tunnel: w320 -> [_ w335 w343 w350 w357 w364 w371 w378 w385 w392]
                  tunnel: w313 -> [_ w329 w337 w344 w351 w358 w365 w372 w379 _]
                  tunnel: w307 -> [_ w328 w336 _ _ _ _ _ _ w386]
                  frame 0, Default {
                  }
                  frame 1 {
                    n178 = global write "总磷总氮断电保存全局变量.vi" "总氮消解时长"(w328) -> ()
                    n179 = global write "总磷总氮断电保存全局变量.vi" "总磷自动测试量程配置"(w329) -> ()
                    n180 = Bundle By Name(cluster=w335, "总磷跨度值"=w333, "总磷零点标准液浓度"=w332, "总磷跨度标准液浓度"=w331, "总磷标准液标准浓度"=w330) -> (w334:T11)
                    n181 = global write "总磷总氮断电保存全局变量.vi" "质控参数设置"(w334) -> ()
                  }
                  frame 2 {
                    n182 = global write "总磷总氮断电保存全局变量.vi" "总氮消解时长"(w336) -> ()
                    n183 = global write "总磷总氮断电保存全局变量.vi" "总氮自动测试量程配置"(w337) -> ()
                    n184 = Bundle By Name(cluster=w343, "总氮跨度值"=w341, "总氮零点标准液浓度"=w340, "总氮跨度标准液浓度"=w339, "总氮标准液标准浓度"=w338) -> (w342:T11)
                    n185 = global write "总磷总氮断电保存全局变量.vi" "质控参数设置"(w342) -> ()
                  }
                  frame 3 {
                    n186 = global write "总磷总氮断电保存全局变量.vi" "氨氮自动测试量程配置"(w344) -> ()
                    n187 = Bundle By Name(cluster=w350, "氨氮跨度值"=w348, "氨氮零点标准液浓度"=w347, "氨氮跨度标准液浓度"=w346, "氨氮标准液标准浓度"=w345) -> (w349:T11)
                    n188 = global write "总磷总氮断电保存全局变量.vi" "质控参数设置"(w349) -> ()
                  }
                  frame 4 {
                    n189 = Bundle By Name(cluster=w357, "磷酸盐跨度值"=w355, "磷酸盐零点标准液浓度"=w354, "磷酸盐跨度标准液浓度"=w353, "磷酸盐标准液标准浓度"=w352) -> (w356:T11)
                    n190 = global write "总磷总氮断电保存全局变量.vi" "磷酸盐自动测试量程配置"(w351) -> ()
                    n191 = global write "总磷总氮断电保存全局变量.vi" "质控参数设置"(w356) -> ()
                  }
                  frame 5 {
                    n192 = global write "总磷总氮断电保存全局变量.vi" "硝氮自动测试量程配置"(w358) -> ()
                    n193 = Bundle By Name(cluster=w364, "硝氮跨度值"=w362, "硝氮零点标准液浓度"=w361, "硝氮跨度标准液浓度"=w360, "硝氮标准液标准浓度"=w359) -> (w363:T11)
                    n194 = global write "总磷总氮断电保存全局变量.vi" "质控参数设置"(w363) -> ()
                  }
                  frame 6 {
                    n195 = Bundle By Name(cluster=w371, "亚硝氮跨度值"=w369, "亚硝氮零点标准液浓度"=w368, "亚硝氮跨度标准液浓度"=w367, "亚硝氮标准液标准浓度"=w366) -> (w370:T11)
                    n196 = global write "总磷总氮断电保存全局变量.vi" "亚硝氮自动测试量程配置"(w365) -> ()
                    n197 = global write "总磷总氮断电保存全局变量.vi" "质控参数设置"(w370) -> ()
                  }
                  frame 7 {
                    n198 = Bundle By Name(cluster=w378, "硅酸盐跨度值"=w376, "硅酸盐零点标准液浓度"=w375, "硅酸盐跨度标准液浓度"=w374, "硅酸盐标准液标准浓度"=w373) -> (w377:T11)
                    n199 = global write "总磷总氮断电保存全局变量.vi" "硅酸盐自动测试量程配置"(w372) -> ()
                    n200 = global write "总磷总氮断电保存全局变量.vi" "质控参数设置"(w377) -> ()
                  }
                  frame 8 {
                    n201 = Bundle By Name(cluster=w385, "硫化物跨度值"=w383, "硫化物零点标准液浓度"=w382, "硫化物跨度标准液浓度"=w381, "硫化物标准液标准浓度"=w380) -> (w384:T11)
                    n202 = global write "总磷总氮断电保存全局变量.vi" "硫化物自动测试量程配置"(w379) -> ()
                    n203 = global write "总磷总氮断电保存全局变量.vi" "质控参数设置"(w384) -> ()
                  }
                  frame 22 {
                    n204 = global write "总磷总氮断电保存全局变量.vi" "CODcr消解时长"(w386) -> ()
                    n205 = Bundle By Name(cluster=w392, "COD跨度值"=w390, "COD零点标准液浓度"=w389, "COD跨度标准液浓度"=w388, "COD标准液标准浓度"=w387) -> (w391:T11)
                    n206 = global write "总磷总氮断电保存全局变量.vi" "质控参数设置"(w391) -> ()
                  }
                }
              }
              frame #1 {
                n207 = call "配置写入.vi"() -> ()  [unwired: 11 in, 1 out]
              }
            }
          }
        }
      }
      event "通讯连接": Value Change {
        n208 = event-data() -> ("NewVal"=w393:bool)  [unwired: 1 in, 5 out]
        n209 = Flush Queue(queue=w394) -> (queue out=w395:refnum<queue>)  [unwired: 1 in, 2 out]
        n210 = case shown="假" w393 {
          tunnel: w395 -> [w396 w398]
          frame False {
            n211 = Enqueue Element(queue=w396, element=cluster{"命令":string, "data":variant} {"命令"="停用模块", "data"=variant} ("元素")) -> ()  [unwired: 2 in, 3 out]
          }
          frame True {
            n212 = Enqueue Element(queue=w398, element=cluster{"命令":string, "data":variant} {"命令"="启用模块", "data"=variant} ("元素")) -> ()  [unwired: 2 in, 3 out]
          }
        }
      }
    }
  }
  n213 = while {
    tunnel: w1 -> [w411]
    tunnel: w3 -> [w410]
    tunnel: w4 -> [w409]
    tunnel: w2 -> [w408]
    stop <- FALSE stop-if-true
    n214 = Wait on Occurrence(2:w408) -> (0:w402:bool)  [unwired: 2 in]
    n215 = flat-sequence {
      tunnel: w411 -> [w418]
      tunnel: w410 -> [w417]
      tunnel: w409 -> [w416]
      tunnel: [w415] -> w405
      tunnel: [w414] -> w404
      tunnel: [w413] -> w403
      tunnel: w402 -> [_]
      frame #0 {
        n216 = property class="Enum (严格)"(reference=w417) -> ("Value"=w414:enum16{"低量程", "高量程"})  [unwired: 1 in, 2 out]
        n217 = property class="Enum (严格)"(reference=w416) -> ("Value"=w413:T1)  [unwired: 1 in, 2 out]
        n218 = property class="Ring (严格)"(reference=w418) -> ("Value"=w415:u16)  [unwired: 1 in, 2 out]
      }
    }
    n219 = flat-sequence {
      tunnel: [w421] -> w407
      tunnel: [w420] -> w406
      tunnel: w405 -> [w419]
      tunnel: w404 -> [w421]
      tunnel: w403 -> [w420]
      tunnel: [w419] -> w400
      tunnel: w407 -> [w430]
      tunnel: w406 -> [w431]
      tunnel: [w424] -> w401
      tunnel: w400 -> [w423]
      tunnel: w401 -> [_]
      frame #0 {
      }
      frame #1 {
        n220 = call "总磷总氮量程读取.vi"("测量参数"=w423) -> ("error out"=w436:errorcluster, "量程参数读取"=w444:T6)  [unwired: 9 in]
        n221 = Unbundle By Name(w444) -> ("测量精度"=→"测量精度":u16, "检出限"=→"检出限":dbl, "上限"=→"量程上限":dbl, "下限"=→"量程下限":dbl, "阈值（低->高）"=→"阈值（低->高）":dbl, "阈值（高->低）"=→"阈值（高->低）":dbl, "稀释度"=→"稀释度":dbl)
        n222 = global read "VAR总磷总氮全局变量.vi" "MB session in"() -> (w422:refnum<class "MB_Master.lvclass">)
        n223 = call "总磷总氮公式读取.vi"("error in (no error)"=w436, "量程"=w430, "测量模式"=w431, "测量参数"=w423) -> ("error out"=w425:errorcluster, "公式"=w435:cluster{"X^2":dbl, "X":dbl, "b":dbl})  [unwired: 6 in]
        n224 = case shown="1, 2, 22" w423 {
          tunnel: [w446 w452] -> w429
          tunnel: [_ w450] -> w428
          tunnel: [w445 w449] -> w427
          tunnel: w425 -> [w445 w448]
          tunnel: w422 -> [w446 w447]
          frame 0, Default {
          }
          frame 1, 2, 22 {
            n225 = call "读取外设配置.vi"("error in (no error)"=w448, "MB session in"=w447) -> ("error out"=w449:errorcluster, "外设配置"=w451:T7, "MB session out"=w452:refnum<class "MB_Master.lvclass">)  [unwired: 7 in]
            n226 = Unbundle By Name(w451) -> ("消解温度下限"=w450:sgl)
          }
        }
        "消解温度" <- w428
        n227 = Unbundle By Name(w435) -> ("X^2"=→"二次多项式系数":dbl, "X"=→"曲线斜率":dbl, "b"=→"曲线截距":dbl)
        n228 = call "盐度补偿值读取.vi"("Error in"=w427, "MB session in"=w429) -> ("error out"=w424:errorcluster, "盐度补偿值"=→"盐度补偿值":sgl)  [unwired: 7 in, 1 out]
      }
      frame #2 {
        n229 = Format Date/Time String() -> (date/time string=→"数据刷新时间":string)  [unwired: 3 in]
      }
    }
  }
  n230 = while {
    tunnel: w1 -> [w456]
    stop <- FALSE stop-if-true
    n231 = property class="Ring (严格)"(reference=w456) -> ("Value"=w455:u16)  [unwired: 1 in, 2 out]
    n232 = global read "总磷总氮断电保存全局变量.vi" "IP"() -> (w473:string)
    n233 = global read "总磷总氮断电保存全局变量.vi" "PORT"() -> (w474:string)
    n234 = Wait (ms)(milliseconds to wait=u32 1000 ("等待时间（毫秒）")) -> ()  [unwired: 1 out]
    n235 = local write "IP"(w473) -> ()
    n236 = global read "总磷总氮断电保存全局变量.vi" "流程路径"() -> (w472:path)
    n237 = local write "PORT"(w474) -> ()
    n238 = global read "总磷总氮断电保存全局变量.vi" "MB通信方式选择"() -> (w470:enum16{"串口", "TCP"})
    n239 = global read "总磷总氮断电保存全局变量.vi" "VISA Resource"() -> (w475:refnum<visa-resource-name>)
    n240 = global read "总磷总氮断电保存全局变量.vi" "盐度自动补偿："() -> (w471:bool)
    n241 = local write "测试流程路径"(w472) -> ()
    n242 = global read "总磷总氮断电保存全局变量.vi" "质控参数设置"() -> (w465:T11)
    n243 = global read "总磷总氮断电保存全局变量.vi" "简易流程路径"() -> (w454:path)
    n244 = local write "通信方式选择"(w470) -> ()
    n245 = local write "请选择串口:"(w475) -> ()
    n246 = local write "盐度自动补偿："(w471) -> ()
    n247 = case shown="1" w455 {
      tunnel: [_ w484 w491 w497 w503 w509 w515 w521 w527 w534] -> w463
      tunnel: [_ w483 w490 _ _ _ _ _ _ w533] -> w464
      tunnel: w465 -> [_ w482 w489 w496 w502 w508 w514 w520 w526 w532]
      tunnel: [_ w481 w488 w495 w501 w507 w513 w519 w525 w531] -> w466
      tunnel: [_ w480 w487 w494 w500 w506 w512 w518 w524 w530] -> w467
      tunnel: [_ w479 w486 w493 w499 w505 w511 w517 w523 w529] -> w468
      tunnel: [_ w478 w485 w492 w498 w504 w510 w516 w522 w528] -> w469
      frame Default {
      }
      frame 1 {
        n248 = Unbundle By Name(w482) -> ("总磷跨度值"=w481:dbl, "总磷零点标准液浓度"=w480:dbl, "总磷跨度标准液浓度"=w479:dbl, "总磷标准液标准浓度"=w478:dbl)
        n249 = global read "总磷总氮断电保存全局变量.vi" "总磷自动测试量程配置"() -> (w484:T13)
        n250 = global read "总磷总氮断电保存全局变量.vi" "总磷消解时长"() -> (w483:dbl)
      }
      frame 2 {
        n251 = Unbundle By Name(w489) -> ("总氮跨度值"=w488:dbl, "总氮零点标准液浓度"=w487:dbl, "总氮跨度标准液浓度"=w486:dbl, "总氮标准液标准浓度"=w485:dbl)
        n252 = global read "总磷总氮断电保存全局变量.vi" "总氮自动测试量程配置"() -> (w491:T13)
        n253 = global read "总磷总氮断电保存全局变量.vi" "总氮消解时长"() -> (w490:dbl)
      }
      frame 3 {
        n254 = Unbundle By Name(w496) -> ("氨氮跨度值"=w495:dbl, "氨氮零点标准液浓度"=w494:dbl, "氨氮跨度标准液浓度"=w493:dbl, "氨氮标准液标准浓度"=w492:dbl)
        n255 = global read "总磷总氮断电保存全局变量.vi" "氨氮自动测试量程配置"() -> (w497:T13)
      }
      frame 4 {
        n256 = Unbundle By Name(w502) -> ("磷酸盐跨度值"=w501:dbl, "磷酸盐零点标准液浓度"=w500:dbl, "磷酸盐跨度标准液浓度"=w499:dbl, "磷酸盐标准液标准浓度"=w498:dbl)
        n257 = global read "总磷总氮断电保存全局变量.vi" "磷酸盐自动测试量程配置"() -> (w503:T13)
      }
      frame 5 {
        n258 = Unbundle By Name(w508) -> ("硝氮跨度值"=w507:dbl, "硝氮零点标准液浓度"=w506:dbl, "硝氮跨度标准液浓度"=w505:dbl, "硝氮标准液标准浓度"=w504:dbl)
        n259 = global read "总磷总氮断电保存全局变量.vi" "硝氮自动测试量程配置"() -> (w509:T13)
      }
      frame 6 {
        n260 = Unbundle By Name(w514) -> ("亚硝氮跨度值"=w513:dbl, "亚硝氮零点标准液浓度"=w512:dbl, "亚硝氮跨度标准液浓度"=w511:dbl, "亚硝氮标准液标准浓度"=w510:dbl)
        n261 = global read "总磷总氮断电保存全局变量.vi" "亚硝氮自动测试量程配置"() -> (w515:T13)
      }
      frame 7 {
        n262 = Unbundle By Name(w520) -> ("硅酸盐跨度值"=w519:dbl, "硅酸盐零点标准液浓度"=w518:dbl, "硅酸盐跨度标准液浓度"=w517:dbl, "硅酸盐标准液标准浓度"=w516:dbl)
        n263 = global read "总磷总氮断电保存全局变量.vi" "硅酸盐自动测试量程配置"() -> (w521:T13)
      }
      frame 8 {
        n264 = Unbundle By Name(w526) -> ("硫化物跨度值"=w525:dbl, "硫化物零点标准液浓度"=w524:dbl, "硫化物跨度标准液浓度"=w523:dbl, "硫化物标准液标准浓度"=w522:dbl)
        n265 = global read "总磷总氮断电保存全局变量.vi" "硫化物自动测试量程配置"() -> (w527:T13)
      }
      frame 22 {
        n266 = Unbundle By Name(w532) -> ("COD跨度值"=w531:dbl, "COD零点标准液浓度"=w530:dbl, "COD跨度标准液浓度"=w529:dbl, "COD标准液标准浓度"=w528:dbl)
        n267 = global read "总磷总氮断电保存全局变量.vi" "COD自动测试量程配置"() -> (w534:T13)
        n268 = global read "总磷总氮断电保存全局变量.vi" "CODcr消解时长"() -> (w533:dbl)
      }
    }
    "消解时长" <- w464
    n269 = local write "简易流程路径"(w454) -> ()
    n270 = local write "跨度值"(w466) -> ()
    n271 = local write "零点核查标液浓度"(w467) -> ()
    n272 = local write "跨度核查标液浓度"(w468) -> ()
    n273 = local write "标样核查标液浓度"(w469) -> ()
    n274 = To Unsigned Word Integer(number=w463) -> (unsigned 16bit integer=w462:T14)
    n275 = Unbundle By Name(w462) -> ("水样测试量程模式"=w461:u16, "空白核查量程模式"=w459:u16, "跨度核查量程模式"=w458:u16, "加标回收量程模式"=w457:u16, "标样核查量程模式"=w460:u16)
    n276 = local write "水样测试量程模式"(w461) -> ()
    n277 = local write "零点核查量程模式"(w459) -> ()
    n278 = local write "跨度核查量程模式"(w458) -> ()
    n279 = local write "加标回收量程模式"(w457) -> ()
    n280 = local write "标样核查量程模式"(w460) -> ()
  }
